vi "Send Message.vi"(8 "error in (no error)":errorcluster, 9 "Message":string, 11 "Communication Clients in":refnum<class "Communication Clients.lvclass">) -> (0 "error out":errorcluster, 3 "Communication Clients out":refnum<class "Communication Clients.lvclass">)   [LabVIEW 2017, in "Communication Clients.lvlib" / "Communication Clients.lvclass"]
uses:
  Communication Clients.lvclass
  Communication Clients.lvclass/Communication Clients.ctl
  src/LabVIEW/vi.lib/BenjaminR/Build Farm/Actors/Communication/WebSocket Client/WebSocket Client Messages/Send Message Msg/Send Message Msg.lvclass/Send Message Msg.ctl
  <vilib>/ActorFramework/Message Enqueuer/Message Enqueuer.lvclass/Message Enqueuer.ctl
  <vilib>/ActorFramework/Message Enqueuer/Enqueue.vi
  src/LabVIEW/vi.lib/BenjaminR/Build Farm/Actors/Communication/WebSocket Client/WebSocket Client Messages/Send Message Msg/Send Message Msg.lvclass
  C:/Program Files (x86)/National Instruments/LabVIEW 2017/vi.lib/ActorFramework/Message/Message.lvclass
  <vilib>/ActorFramework/Message Priority Queue/Priority Enqueue.vi
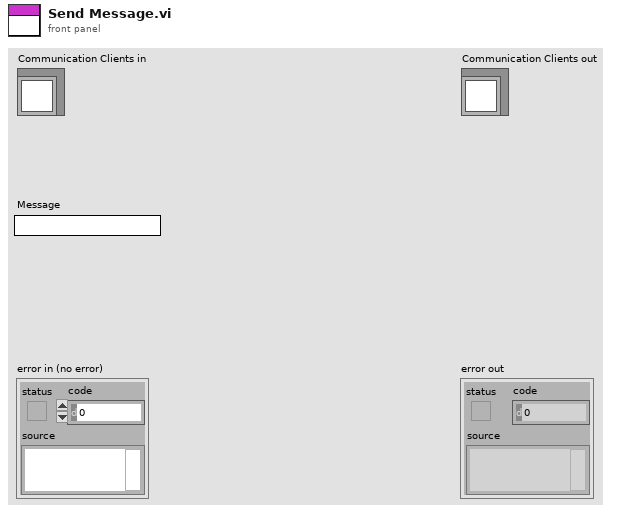
[diagram p1: front panel]
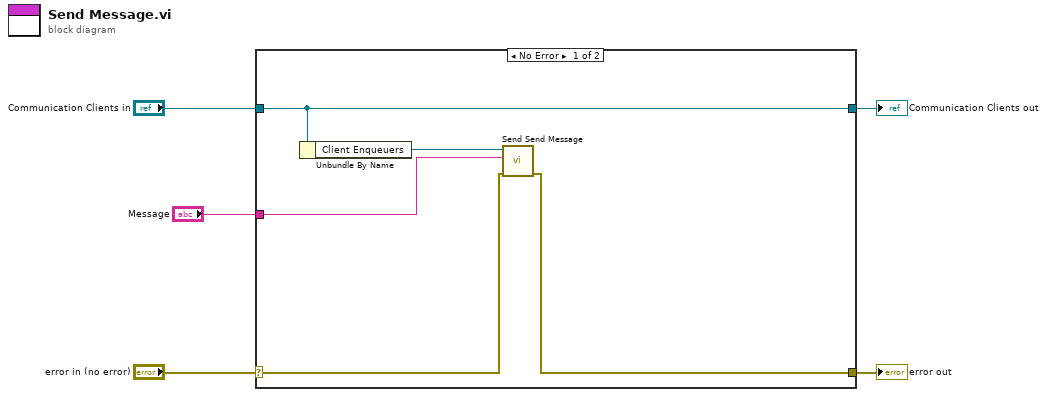
[diagram p0: block diagram]
diagram:
  n1 = case shown="No Error" "error in (no error)" {
    selector: "error in (no error)" -> [w9 w12]
    tunnel: [w8 w12] -> w4
    tunnel: [w10 w11] -> w2
    tunnel: "Communication Clients in" -> [w10 w11]
    tunnel: "Message" -> [w6 _]
    frame No Error {
      n2 = Unbundle By Name(w10) -> ("Client Enqueuers"=w7:refnum<class "Message Enqueuer.lvclass">)
      n3 = call "Send Send Message.vi"("error in (no error)"=w9, "Message"=w6, "Message Enqueuer in"=w7) -> ("error out"=w8:errorcluster)  [unwired: 7 in, 1 out]
    }
    frame Error {
    }
  }
  "error out" <- w4
  "Communication Clients out" <- w2
